vi "modbus reg to real.vi"(8 "Error In":errorcluster, 9 "Reg":dbl, 10 "Scale Min range":dbl, 11 "Scale Max Range":dbl) -> (0 "Error Out":errorcluster, 2 "output":dbl)   [LabVIEW 2016, in "Modbus-Instr.lvclass"]
uses:
  Modbus-Instr_class/Modbus-Instr.lvclass
panel:
  # "Formula node to calc the modbus Reg \nto real numbers.\nin the Adam 4000/5000 range modules."
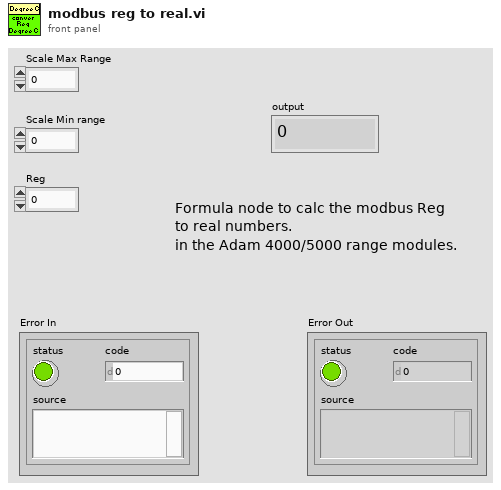
[diagram p1: front panel]
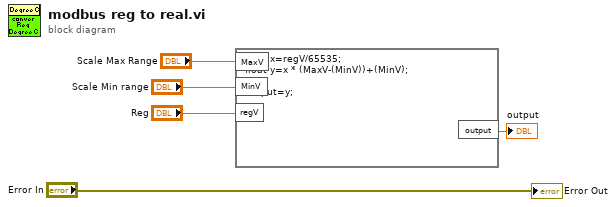
[diagram p0: block diagram]
diagram:
  n1 = formula code="float x=regV/65535;\nfloat y=x * (MaxV-(MinV))+(MinV);\n\noutput=y;"("MaxV"="Scale Max Range", "MinV"="Scale Min range", "regV"="Reg") -> ("output"=→"output":dbl)
  "Error Out" <- "Error In"
